vi "BCtr_Wt.vi"(9 "N_NAB":i32, 10 "NB":u16[](array[numeric])=[80, 1], 11 "NA":u16[](array[numeric])=[1, 220]) -> (0 "W":dbl[](array[numeric]), 3 "T\nT":dbl[](array[numeric]))   [LabVIEW 2016]
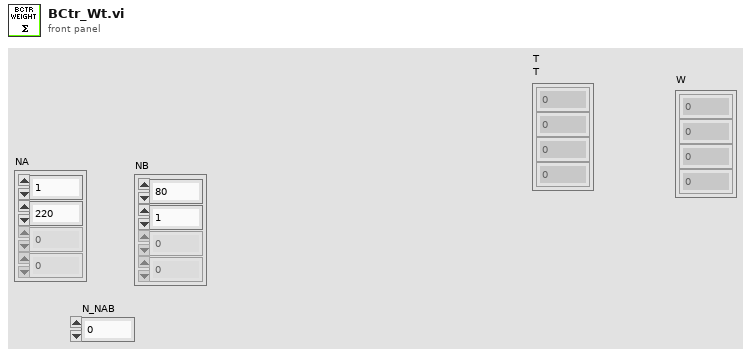
[diagram p1: front panel]
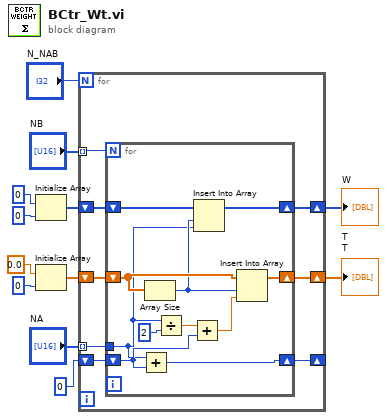
[diagram p0: block diagram]
diagram:
  n1 = Initialize Array(0, 0) -> (w2:i32[])
  n2 = Initialize Array(0.0, 0) -> (w6:dbl[])
  n3 = for {
    N: "N_NAB" -> [_]
    tunnel: "NA" -> [w18] mode=indexing
    tunnel: "NB" -> [w20] mode=indexing
    shift-right: [w17] -> _
    shift-left: 0 -> [w19]
    shift-right: [w15] -> w9
    shift-left: w6 -> [w16]
    shift-right: [w13] -> w1
    shift-left: w2 -> [w14]
    n4 = for {
      N: w20 -> [_]
      shift-right: [w31] -> w17
      shift-left: w19 -> [w25]
      tunnel: w18 -> [w22]
      shift-right: [w26] -> w15
      shift-left: w16 -> [w28]
      shift-right: [w21] -> w13
      shift-left: w14 -> [w24]
      n5 = Add(x=w22, y=w25) -> (x+y=w31:i32)
      n6 = Array Size(array=w28) -> (size(s)=w23:i32)
      n7 = Divide(x=w22, y=2) -> (x/y=w29:dbl)
      n8 = Add(x=w29, y=w25) -> (x+y=w27:dbl)
      n9 = Insert Into Array(array=w24, index=w23, new element=w22) -> (w21:i32[])
      n10 = Insert Into Array(array=w28, index=w23, new element=w27) -> (w26:dbl[])
    }
  }
  "T\nT" <- w9
  "W" <- w1
